vi "write_files_01.vi"(0 "connection ID IN":refnum<k5>, 1 "Path":path, 3 "error in":errorcluster, 4 "FileFlag (d v)":string="d") -> (5 "connection ID Out":refnum<k5>, 7 "error out":errorcluster)   [LabVIEW 2010]
panel:
  out "NTimes":i32
  out "Size":i32
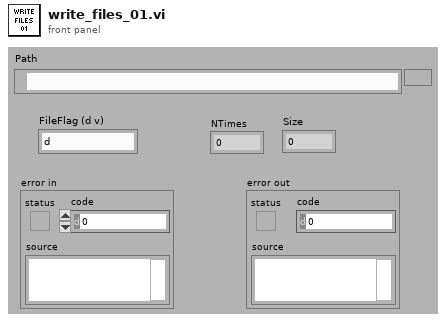
[diagram p1: front panel]
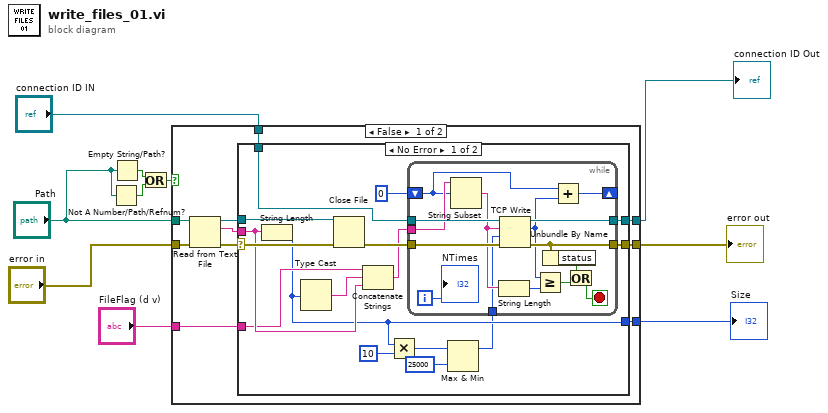
[diagram p0: block diagram]
diagram:
  n1 = Not A Number/Path/Refnum?(number/path/refnum="Path") -> (NaN/Path/Refnum?=w2:bool)
  n2 = Empty String/Path?(string/path="Path") -> (empty?=w3:bool)
  n3 = Or(x=w3, y=w2) -> (x .or. y?=w1:bool)
  n4 = case shown="False" w1 {
    tunnel: [w20 w54] -> w10
    tunnel: "error in" -> [w19 w54]
    tunnel: [w18 w55] -> w8
    tunnel: "connection ID IN" -> [w17 w55]
    tunnel: [w13 _] -> w6
    tunnel: "Path" -> [w12 _]
    tunnel: "FileFlag (d v)" -> [w11 _]
    frame False {
      n5 = Read from Text File(file (use dialog)=w12, error in=w19) -> (refnum out=w15:refnum<file>, text=w14:string, error out=w16:errorcluster)  [unwired: 2 in, 1 out]
      n6 = case shown="No Error" w16 {
        selector: w16 -> [w36 w53]
        tunnel: [w29 w53] -> w20
        tunnel: w15 -> [w35 _]
        tunnel: w17 -> [w33 w52]
        tunnel: [w28 w52] -> w18
        tunnel: [w25 _] -> w13
        tunnel: w14 -> [w31 _]
        tunnel: w11 -> [w30 _]
        frame No Error {
          n7 = String Length(string=w31) -> (length=w25:i32)
          n8 = Type Cast(x=w25) -> (*(type *) &x=w34:string)  [unwired: 1 in]
          n9 = Close File(refnum=w35, error in=w36) -> (error out=w32:errorcluster)  [unwired: 1 out]
          n10 = Concatenate Strings(w30, w34, w31) -> (w26:string)
          n11 = Multiply(x=w25, y=10) -> (x*y=w22:i32)
          n12 = Max & Min(x=w22, y=25000 ("timeout ms (25000)")) -> (max(x,y)=w21:i32)  [unwired: 1 out]
          n13 = while {
            tunnel: w33 -> [w51]
            tunnel: w32 -> [w50]
            tunnel: w26 -> [w48]
            tunnel: [w45] -> w29
            tunnel: [w49] -> w28
            shift-right: [w39] -> _
            shift-left: 0 ("bytes written") -> [w40]
            tunnel: w21 -> [w37]
            i -> [w38]
            stop <- w42 stop-if-true
            n14 = String Subset(string=w48, offset (0)=w40) -> (substring=w47:string)  [unwired: 1 in]
            n15 = String Length(string=w47) -> (length=w46:i32)
            n16 = TCP Write(connection ID=w51, data in=w47, error in (no error)=w50, 9:w37) -> (connection ID out=w49:refnum<k5>, bytes written=w41:i32, error out=w45:errorcluster)
            n17 = Greater Or Equal?(x=w41, y=w46) -> (x >= y?=w44:bool)
            n18 = Unbundle By Name(w45) -> ("status"=w43:bool)
            n19 = Add(x=w40, y=w41) -> (x+y=w39:i32)
            n20 = Or(x=w43, y=w44) -> (x .or. y?=w42:bool)
            "NTimes" <- w38
          }
        }
        frame Error {
        }
      }
    }
    frame True {
    }
  }
  "error out" <- w10
  "connection ID Out" <- w8
  "Size" <- w6
